vi "WaitForInit.vi"(8 "error in (no error)":errorcluster, 11 "Connection in":refnum<class "Connection.lvclass">) -> (0 "error out":errorcluster, 3 "Connection out":refnum<class "Connection.lvclass">)   [LabVIEW 2022 SP3, in "Connection.lvlib" / "Connection.lvclass"]
uses:
  Connection.lvclass
  C:/Program Files (x86)/National Instruments/LabVIEW 2022/vi.lib/ActorFramework/Actor/Actor.lvclass
  Connection.lvclass/Connection.ctl
  <vilib>/ActorFramework/Actor/Actor.lvclass/Actor.ctl
  <vilib>/ActorFramework/Message Enqueuer/Message Enqueuer.lvclass/Message Enqueuer.ctl
  <vilib>/ActorFramework/Message Enqueuer/Init from Existing Queue.vi
  <vilib>/ActorFramework/Message Enqueuer/Enqueue.vi
  Connection Messages/WaitForInit Msg/WaitForInit Msg.lvclass
  C:/Program Files (x86)/National Instruments/LabVIEW 2022/vi.lib/ActorFramework/Message/Message.lvclass
  Connection Messages/Kill Msg/Kill Msg.lvclass
  <vilib>/ActorFramework/Message Priority Queue/Priority Enqueue.vi
  <vilib>/ActorFramework/Message Enqueuer/Message Enqueuer.lvclass
  <vilib>/ActorFramework/Actor/Actor.lvclass
  C:/Users/jakub/repos/gh/lv-cli-example/Source/Connection/Connection/Connection.lvclass
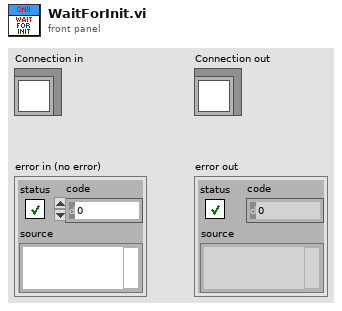
[diagram p1: front panel]
types:
  T1 = typedef "Connection.lvlib/Connection.lvclass/_State.ctl" = enum16{"WaitForInit", "Active", "Dying"}
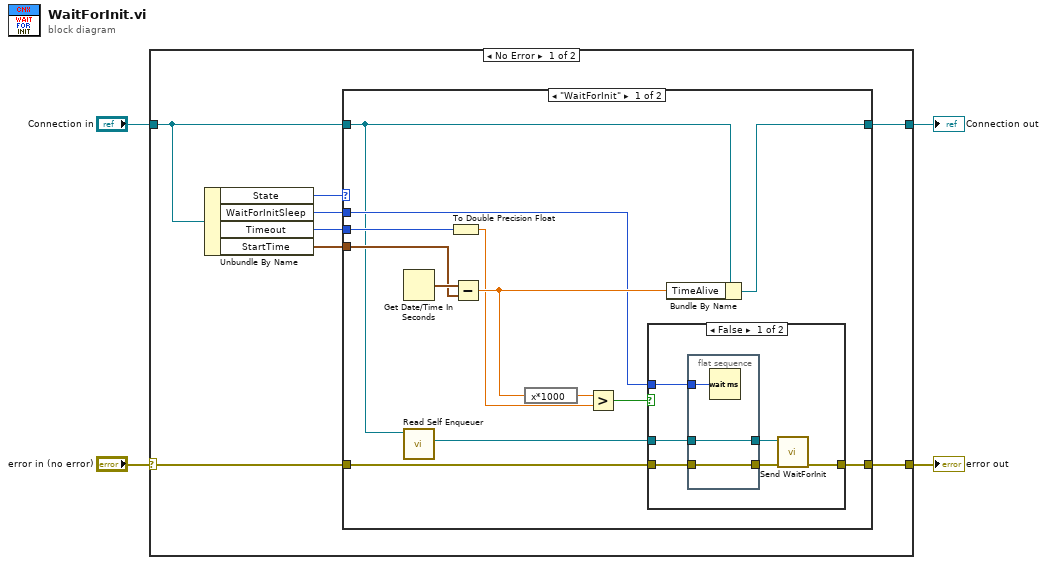
[diagram p0: block diagram]
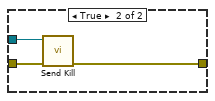
[diagram p2: hidden frame]
diagram:
  n1 = case shown="No Error" "error in (no error)" {
    selector: "error in (no error)" -> [w9 w41]
    tunnel: [w8 w41] -> w3
    tunnel: [w11 w40] -> w1
    tunnel: "Connection in" -> [w5 w40]
    frame No Error {
      n2 = Unbundle By Name(w5) -> ("State"=w6:T1, "WaitForInitSleep"=w7:u32, "Timeout"=w10:i32, "StartTime"=w12:timestamp)
      n3 = case shown="\"WaitForInit\"" w6 {
        tunnel: w12 -> [w24 _]
        tunnel: [w23 w39] -> w11
        tunnel: w10 -> [w21 _]
        tunnel: w9 -> [w19 w38]
        tunnel: [w18 w38] -> w8
        tunnel: w5 -> [w14 w39]
        tunnel: w7 -> [w15 _]
        frame "WaitForInit" {
          n4 = Get Date/Time In Seconds() -> (seconds since 1Jan1904=w25:timestamp)
          n5 = call <vilib>:"Read Self Enqueuer.vi"("Actor"=w14) -> ("Self Enqueuer"=w16:refnum<class "Message Enqueuer.lvclass">)  [unwired: 10 in]
          n6 = To Double Precision Float(number=w21) -> (double precision float=w20:dbl)
          n7 = Subtract(x=w25, y=w24) -> (x-y=w22:dbl)
          n8 = expression code="x*1000"(w22) -> (w13:dbl)
          n9 = Greater?(x=w13, y=w20) -> (0:w17:bool)
          n10 = case shown="False" w17 {
            tunnel: [w31 w37] -> w18
            tunnel: w19 -> [w29 w36]
            tunnel: w16 -> [w28 w35]
            tunnel: w15 -> [w30 _]
            frame False {
              n11 = flat-sequence {
                tunnel: w30 -> [w34]
                tunnel: w29 -> [w32]
                tunnel: w28 -> [w33]
                tunnel: [w33] -> w27
                tunnel: [w32] -> w26
                frame #0 {
                  n12 = Wait (ms)(milliseconds to wait=w34) -> ()  [unwired: 1 out]
                }
              }
              n13 = call "Send WaitForInit.vi"("error in (no error)"=w26, "Message Enqueuer"=w27) -> ("error out"=w31:errorcluster)  [unwired: 8 in, 1 out]
            }
            frame True {
              n14 = call "Send Kill.vi"("error in (no error)"=w36, "Message Enqueuer"=w35) -> ("error out"=w37:errorcluster)  [unwired: 8 in, 1 out]
            }
          }
          n15 = Bundle By Name(cluster=w14, "TimeAlive"=w22) -> (w23:refnum<class "Connection.lvclass">)
        }
        frame Default {
        }
      }
    }
    frame Error {
    }
  }
  "error out" <- w3
  "Connection out" <- w1
